vi "Image_Slider.vi"() -> ()   [LabVIEW 2016]
panel:
  out "2D Picture":picture
  in  "Folder of Images":path
  in  "Timeout":i32=100
  in  "Slide through your images":i32(slide) max=101 scale=0.0..100.0
  in  "OK":bool
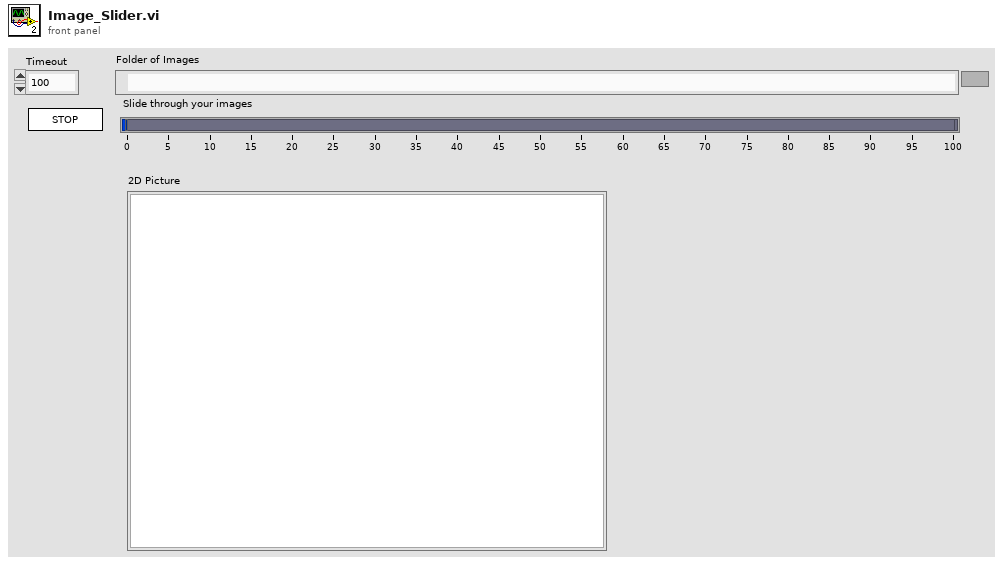
[diagram p1: front panel]
types:
  T1 = enum32{"invalid app kind", "Development System", "Run Time System", "Student Edition", "Embedded LabVIEW", "Evaluation", "Custom"}
  T2 = enum32{"Invalid", "Standard", "Closed", "Hidden", "Minimized", "Maximized"}
  T3 = cluster{"Core":cluster{"Current VI Reference":refnum<vi>, "Close Panel on Exit?":bool}, "Your Boolean data":bool, "Your string data":string, picture[], "individual picture":picture, "Folder of Images":path, i32, i32}
  T4 = cluster{"Current VI Reference":refnum<vi>, "Close Panel on Exit?":bool}
  T5 = typedef "imagedata.ctl" = cluster{"image type":i32, "image depth":i32, "image":u8[], "mask":u8[], "colors":u32[], "Rectangle":cluster{"left":i16, "top":i16, "right":i16, "bottom":i16}}
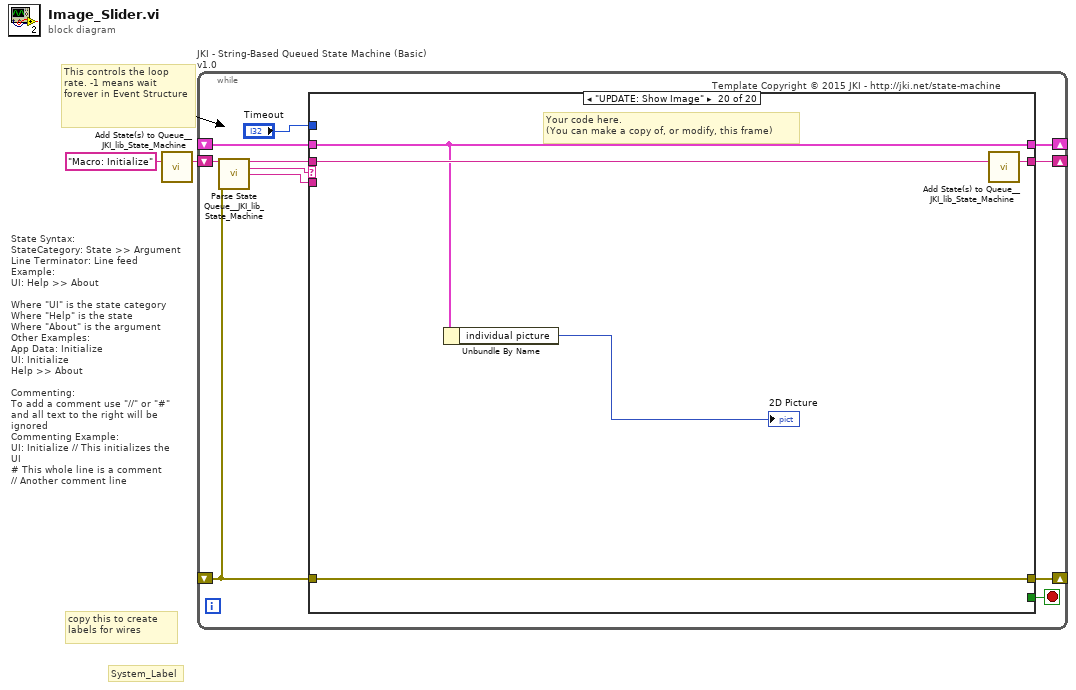
[diagram p0: block diagram]
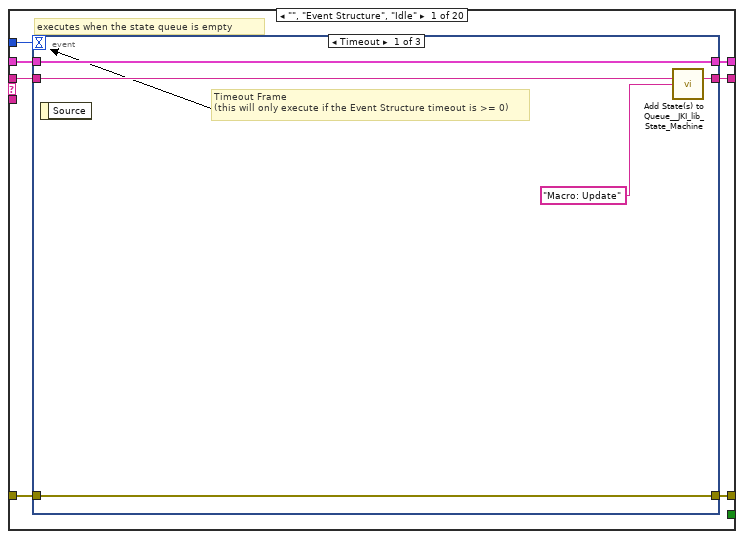
[diagram p2: hidden frame]
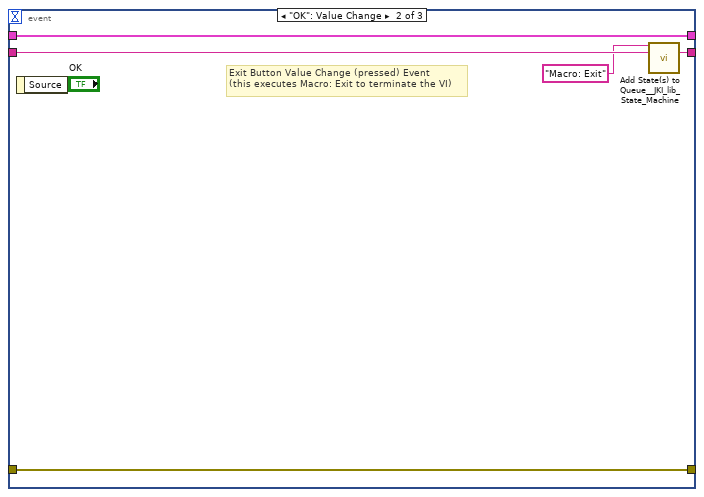
[diagram p3: hidden frame]
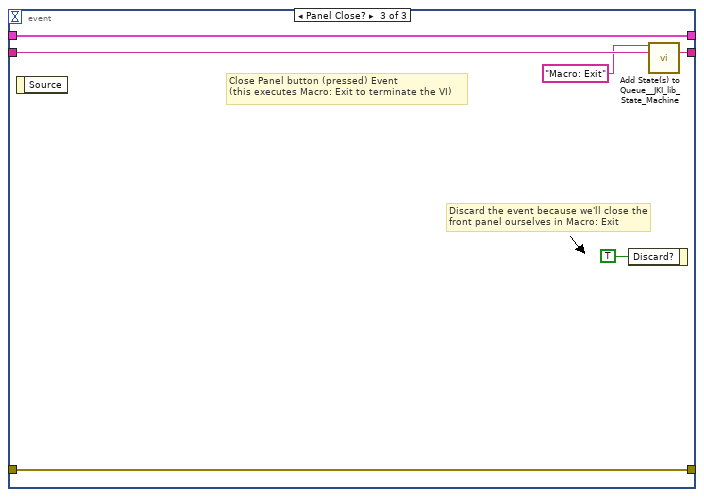
[diagram p4: hidden frame]
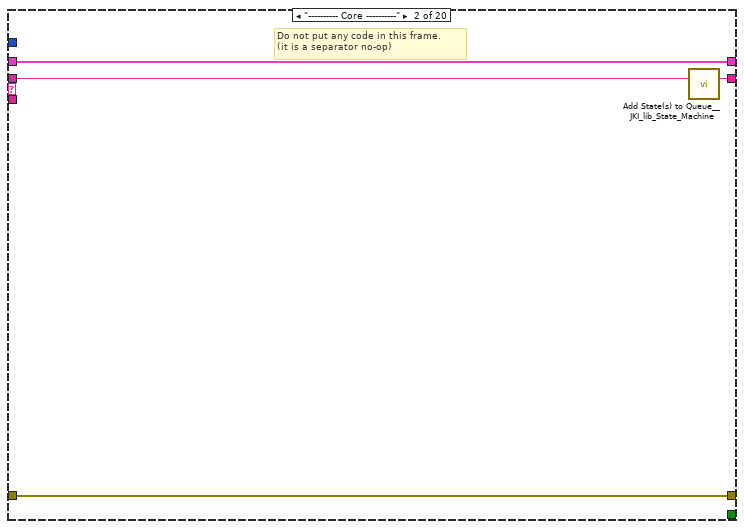
[diagram p5: hidden frame]
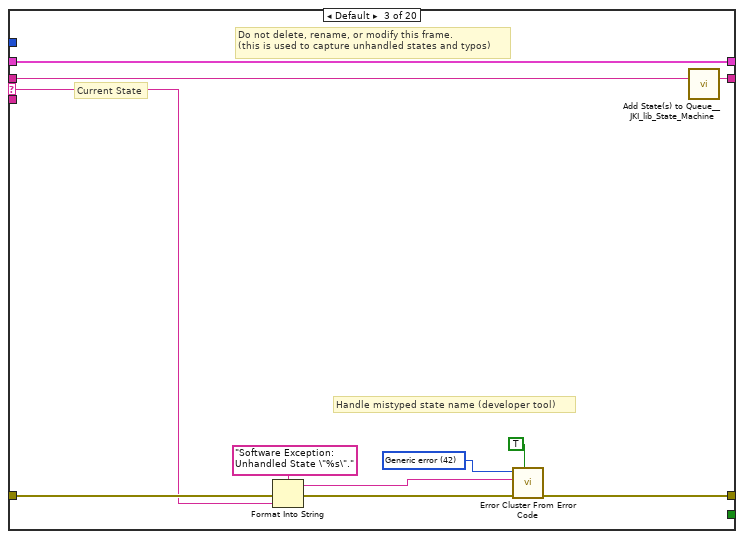
[diagram p6: hidden frame]
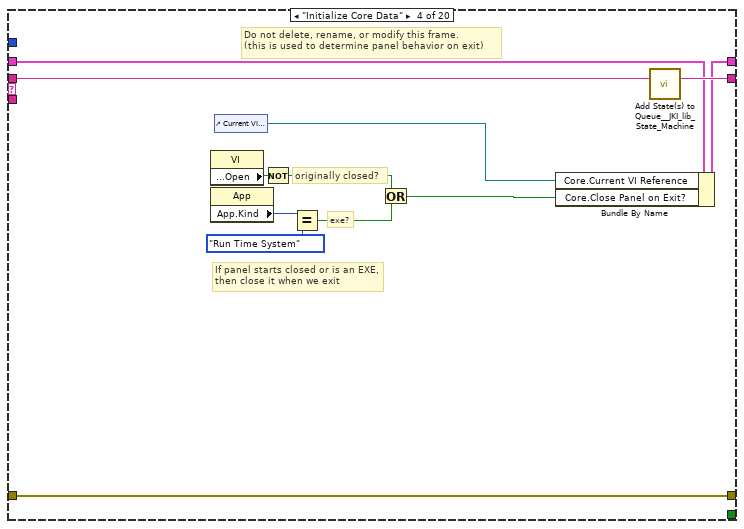
[diagram p7: hidden frame]
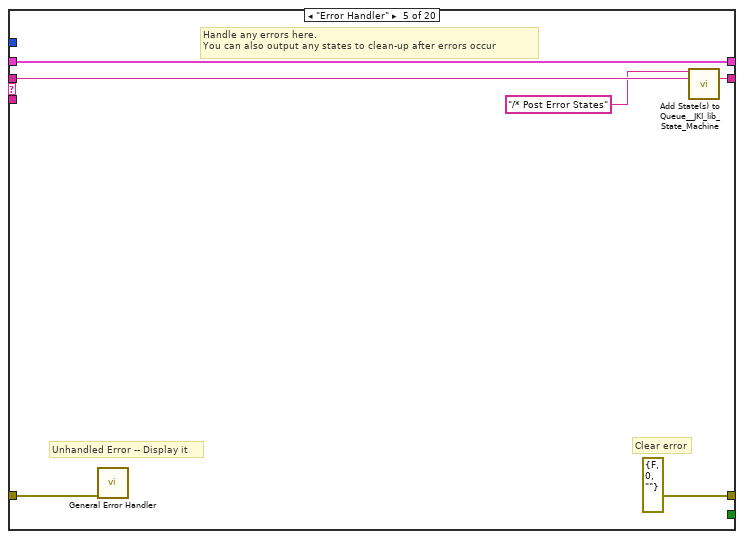
[diagram p8: hidden frame]
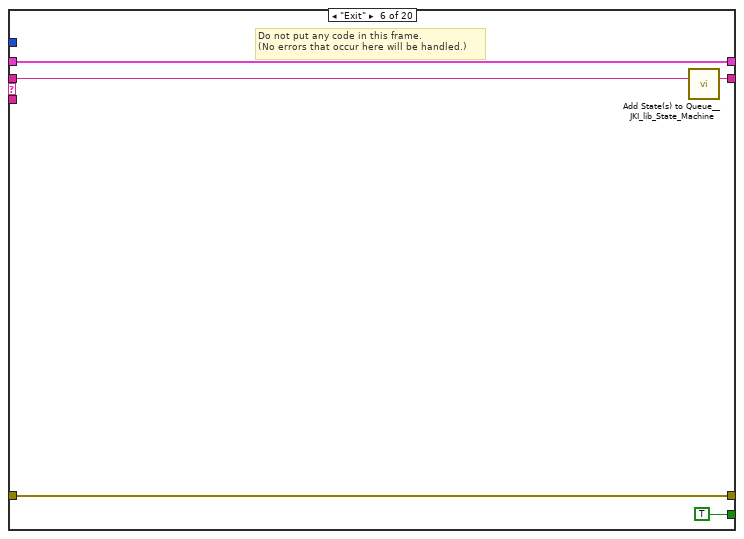
[diagram p9: hidden frame]
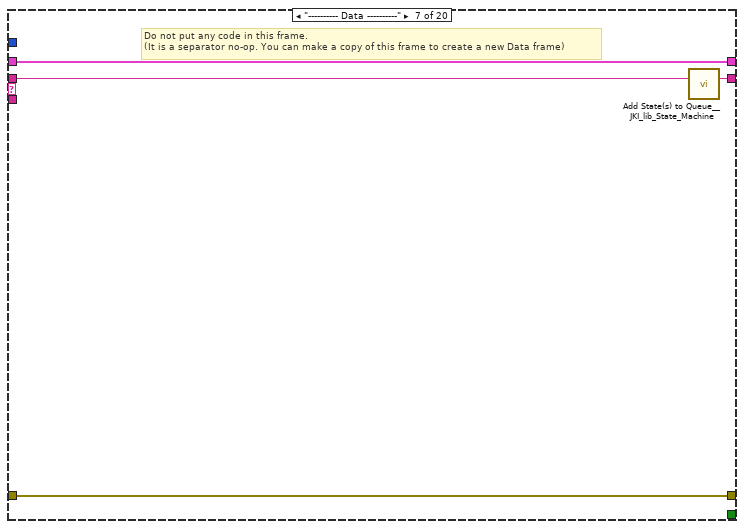
[diagram p10: hidden frame]
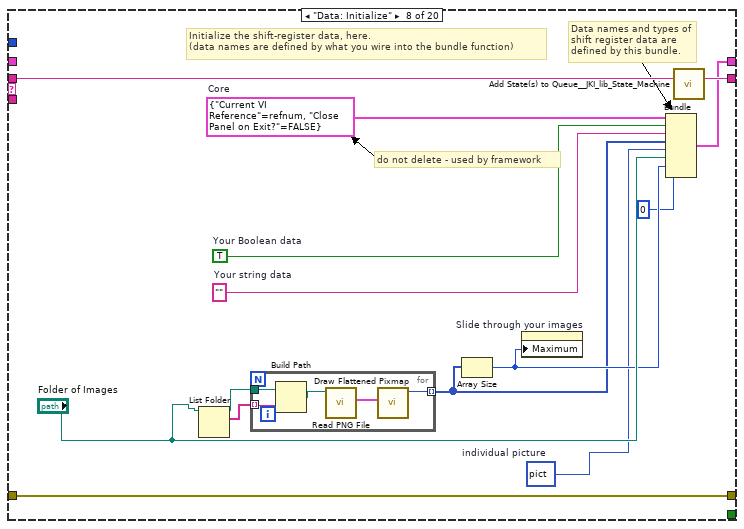
[diagram p11: hidden frame]
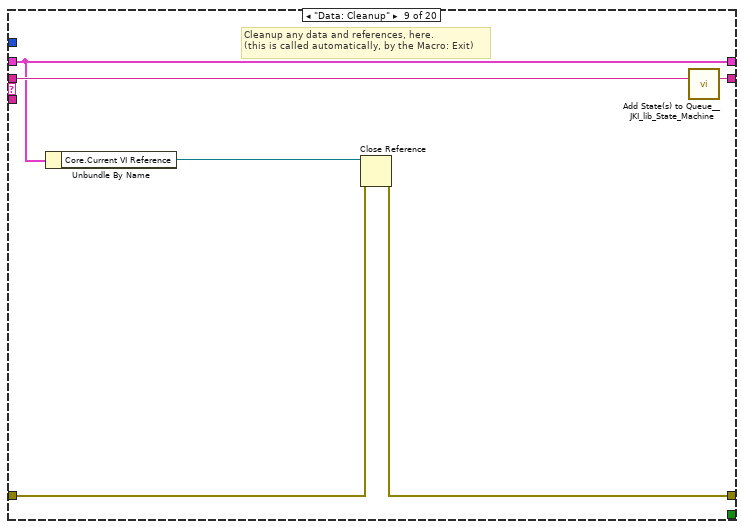
[diagram p12: hidden frame]
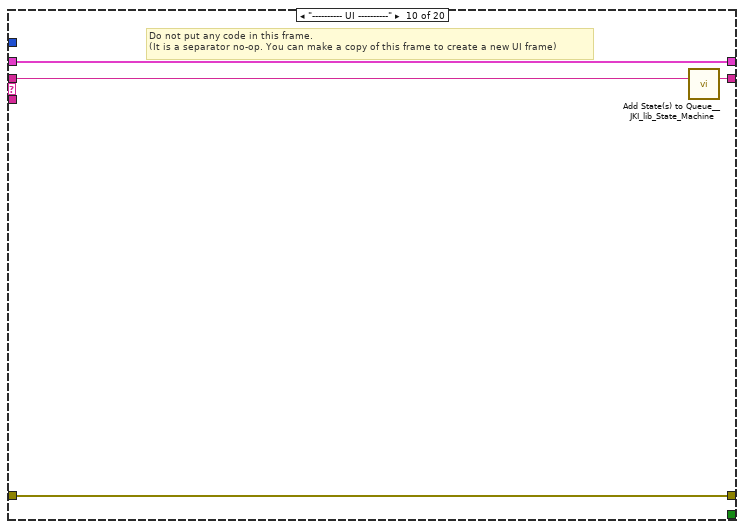
[diagram p13: hidden frame]
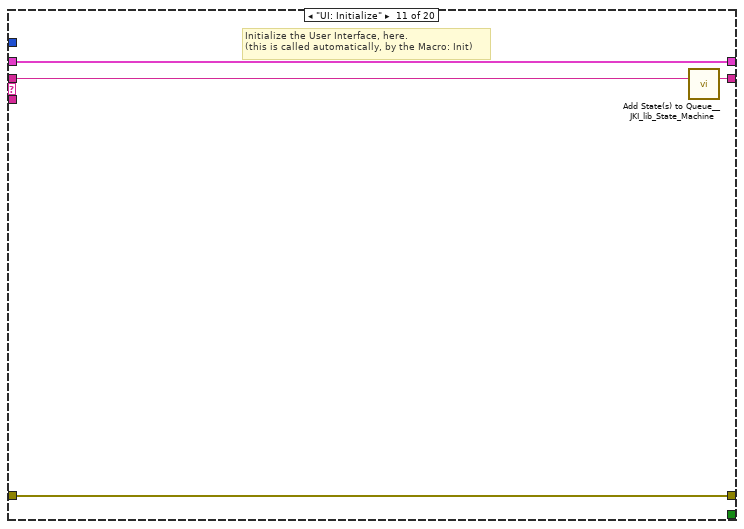
[diagram p14: hidden frame]
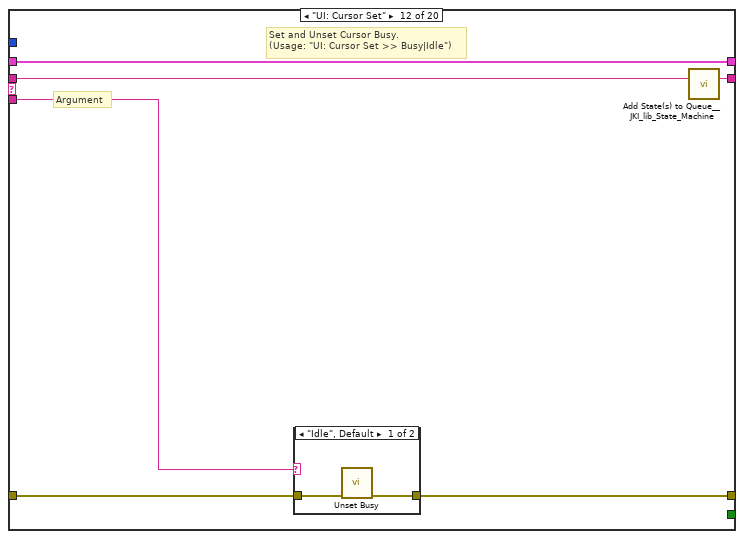
[diagram p15: hidden frame]
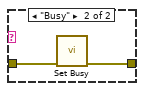
[diagram p16: hidden frame]
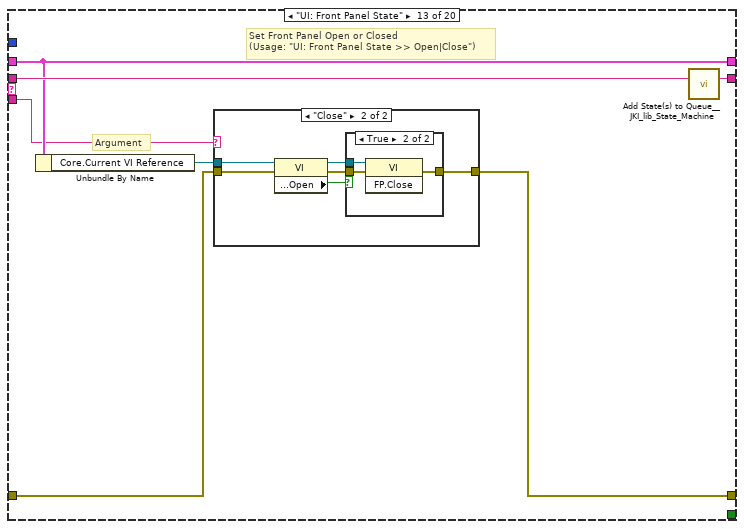
[diagram p17: hidden frame]
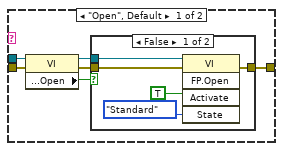
[diagram p18: hidden frame]
diagram:
  # "State Syntax:\nStateCategory: State >> Argument\nLine Terminator: Line feed\nExample:\nUI: Help >> About\n\nWhere \"UI\" is the state category\nWhere \"Help\" is the state\nWhere \"About\" is the argument\nOther Examples:\nApp Data: Initialize\nUI: Initialize\nHelp >> About\n\nCommenting:\nTo add a comment use \"//\" or \"#\" and all text to the right will be ignored\nCommenting Example:\nUI: Initialize // This initializes the UI\n# This whole line is a comment\n// Another comment line"
  # "copy this to create labels for wires"
  # "This controls the loop rate. -1 means wait forever in Event Structure"
  # "System_Label"
  n1 = call <vilib>:"Add State(s) to Queue__JKI_lib_State_Machine.vi"("State(s) in (\"\")"="Macro: Initialize") -> ("States Out"=w2:string)  [unwired: 14 in]
  n2 = while "JKI - String-Based Queued State Machine (Basic) v1.0" {
    shift-right: [w6] -> _
    shift-left: _ -> [w5]
    shift-right: [w9] -> _
    shift-left: _ -> [w3]
    shift-right: [w8] -> _
    shift-left: w2 -> [w10]
    stop <- w7 stop-if-true
    # "Template Copyright © 2015 JKI - http://jki.net/state-machine"
    n3 = call <vilib>:"Parse State Queue__JKI_lib_State_Machine.vi"("State Queue"=w10, "Error In (no error)"=w3) -> ("Remaining States"=w12:string, "Current State"=w13:string, "Arguments"=w11:string)  [unwired: 11 in]
    n4 = case shown="\"UPDATE: Show Image\"" w13 {
      selector: w13 -> [_ _ w41 _ _ _ _ _ _ _ _ _ _ _ _ _ _ _ _ _]
      tunnel: w12 -> [w20 w40 w45 w63 w69 w74 w78 w92 w103 w107 w111 w117 w128 w154 w159 w169 w174 w178 w186 w191]
      tunnel: w11 -> [_ _ _ _ _ _ _ _ _ _ _ w112 w122 _ _ _ _ _ _ _]
      tunnel: w5 -> [w18 w37 w43 w54 w66 w72 w75 _ w98 w104 w109 w115 w124 w151 w156 w166 w171 w175 w181 w188]
      tunnel: [w17 w38 w47 w60 errorcluster {"status"=FALSE, "code"=0, "source"=""} ("error out") w71 w76 w89 w99 w105 w108 w113 w125 w152 w157 w167 w172 w176 w184 w189] -> w9
      tunnel: w3 -> [w16 w38 w46 w60 w65 w71 w76 w89 w100 w105 w108 w114 w126 w152 w157 w167 w172 w176 w184 w189]
      tunnel: [w19 w39 w44 w62 w68 w73 w77 w91 w102 w106 w110 w116 w127 w153 w158 w168 w173 w177 w185 w190] -> w8
      tunnel: [_ _ _ _ _ TRUE _ _ _ _ _ _ _ _ _ _ _ _ _ _] -> w7
      tunnel: [w15 w37 w43 w61 w66 w72 w75 w90 w98 w104 w109 w115 w124 w151 w156 w166 w171 w175 w182 w188] -> w6
      tunnel: "Timeout" -> [w14 _ _ _ _ _ _ _ _ _ _ _ _ _ _ _ _ _ _ _]
      frame "", "Event Structure", "Idle" {
        # "executes when the state queue is empty"
        n5 = event shown="[0] Timeout" {
          selector: _ -> [_ _ _]
          dyn-events: _ -> [_ _ _]
          timeout: w14 -> [_ _ _]
          tunnel: w20 -> [w25 w30 w36]
          tunnel: [w24 w29 w35] -> w19
          tunnel: w18 -> [w22 w27 w33]
          tunnel: [w23 w28 w34] -> w17
          tunnel: w16 -> [w23 w28 w34]
          tunnel: [w22 w27 w33] -> w15
          event Timeout {
            # "Timeout Frame\n(this will only execute if the Event Structure timeout is >= 0)"
            n6 = event-data() -> ()  [unwired: 1 in, 1 out]
            n7 = call <vilib>:"Add State(s) to Queue__JKI_lib_State_Machine.vi"("State(s) in (\"\")"=w25, "State(s) at Back (\"\")"="Macro: Update" ("State(s) at Back (\"\")")) -> ("States Out"=w24:string)  [unwired: 13 in]
          }
          event "OK": Value Change {
            # "Exit Button Value Change (pressed) Event\n(this executes Macro: Exit to terminate the VI)"
            n8 = event-data() -> ()  [unwired: 1 in, 1 out]
            n9 = call <vilib>:"Add State(s) to Queue__JKI_lib_State_Machine.vi"("State(s) in Front (\"\")"="Macro: Exit", "State(s) in (\"\")"=w30) -> ("States Out"=w29:string)  [unwired: 13 in]
          }
          event Panel Close? {
            # "Discard the event because we'll close the front panel ourselves in Macro: Exit"
            # "Close Panel button (pressed) Event\n(this executes Macro: Exit to terminate the VI)"
            n10 = event-data() -> ()  [unwired: 1 in, 1 out]
            n11 = event-data("Discard?"=TRUE) -> ()  [unwired: 1 in, 1 out]
            n12 = call <vilib>:"Add State(s) to Queue__JKI_lib_State_Machine.vi"("State(s) in Front (\"\")"="Macro: Exit", "State(s) in (\"\")"=w36) -> ("States Out"=w35:string)  [unwired: 13 in]
          }
        }
      }
      frame "---------- Core ----------" {
        # "Do not put any code in this frame.\n(it is a separator no-op)"
        n13 = call <vilib>:"Add State(s) to Queue__JKI_lib_State_Machine.vi"("State(s) in (\"\")"=w40) -> ("States Out"=w39:string)  [unwired: 14 in]
      }
      frame Default {
        w50 = 42 items=["No error", "Argument error", "Memory is full", "Out of zone", "End of file", "File already open", "Generic file I/O error", "File not found", "File permission error", "Disk is full", "Duplicate path", "Too many files open", "System feature not enabled", "Resource file not found", "Cannot add resource", "Resource not found", "Image not found", "Image memory error", "Pen does not exist", "Config type invalid", "Config token not found", "Config parse error", "Config memory error", "Bad external code format", "Bad external code offset", "External code not present", "Null window", "Destroy window error", "Null menu", "Print aborted", "Bad print record", "Print driver error", "Windows error during printing", "Memory error during printing", "Print dialog error", "Generic print error", "Invalid device refnum", "Device not found", "Device parameter error", "Device unit error", "Cannot open device", "Device call aborted", "Generic error", "Cancelled by user", "Object ID too low", "Object ID too high", "Object not in heap", "Unknown heap", "Unknown object (invalid DefProc)", "Unknown object (DefProc not in table)", "Message out of range", "Invalid (null) method", "Unknown message", "Manager call not supported", "Bad address", "Network operation in progress", "Network operation timed out", "Connection is busy", "Network attribute not supported", "Network error", "Address in use", "System out of memory", "Connection aborted", "Connection refused", "Not connected", "Already connected", "Connection closed", "Initialization error (interapplication manager)", "Bad occurrence", "Wait on unbound occurrence handler", "Occurrence queue overflow", "Datalog type conflict", "Unused", "Unrecognized type (interapplication manager)", "Memory corrupt", "Failed to make temporary DLL", "Old CIN version", "Drag socket not found", "Failed to load drop-object", "Failed to register OLE object", "Failed to release OLE object", "Format specifier type mismatch", "Unknown format specifier", "Too few format specifiers", "Too many format specifiers", "Scan failed", "Newer CIN version", "Error converting to variant", "Runtime menu error", "Password tampered", "Variant attribute not found", "Incompatible variant data type", "Event data is not available", "Event Store is not present", "Occurrence is not found", "Event Queue is not created", "Event info is not available", "Refnum passed is NULL", "Error retrieving Class GUID", "Error retrieving CoClass GUID", "Error retrieving TypeLib GUID.", "Bad built application magic bytes.", "Specific driver is different from the specific driver associated with the Logical Name.", "There is no session opened to the class driver.", "Max Error", "MAX - Error with config objects", "MAX - Error loading configuration", "MAX - Group not supported"]
        # "Current State"
        # "Do not delete, rename, or modify this frame.\n(this is used to capture unhandled states and typos)"
        # "Handle mistyped state name (developer tool)"
        n14 = Format Into String(format string="Software Exception: Unhandled State \"%s\"." ("message"), error in=w46, w41) -> (resulting string=w49:string, error out=w48:errorcluster)  [unwired: 1 in]
        n15 = call <vilib>:"Error Cluster From Error Code.vi"("show call chain? (False)"=TRUE, "error in (no error)"=w48, "error message (\"\")"=w49, "error code (0)"=w50) -> ("error out"=w47:errorcluster)  [unwired: 5 in]
        n16 = call <vilib>:"Add State(s) to Queue__JKI_lib_State_Machine.vi"("State(s) in (\"\")"=w45) -> ("States Out"=w44:string)  [unwired: 14 in]
      }
      frame "Initialize Core Data" {
        # "Do not delete, rename, or modify this frame.\n(this is used to determine panel behavior on exit)"
        # "originally closed?"
        # "exe?"
        # "If panel starts closed or is an EXE, then close it when we exit"
        n17 = property class="VI"() -> ("Front Panel.Open"=w59:bool)  [unwired: 2 in, 2 out]
        n18 = property class="App"() -> ("App.Kind"=w58:T1)  [unwired: 2 in, 2 out]
        n19 = control-ref of="Current VI Reference"() -> (w52:refnum<vi>)
        n20 = Not(x=w59) -> (.not. x?=w56:bool)
        n21 = Equal?(x=w58, y=T1."Run Time System" ("Application:Kind")) -> (x = y?=w55:bool)
        n22 = Or(x=w56, y=w55) -> (x .or. y?=w53:bool)
        n23 = Bundle By Name(cluster=w54, "Core.Current VI Reference"=w52, "Core.Close Panel on Exit?"=w53) -> (w61:T3)
        n24 = call <vilib>:"Add State(s) to Queue__JKI_lib_State_Machine.vi"("State(s) in (\"\")"=w63) -> ("States Out"=w62:string)  [unwired: 14 in]
      }
      frame "Error Handler" {
        # "Unhandled Error -- Display it"
        # "Handle any errors here.\nYou can also output any states to clean-up after errors occur"
        # "Clear error"
        n25 = call <vilib>:"General Error Handler.vi"("error in (no error)"=w65) -> ()  [unwired: 10 in, 5 out]
        n26 = call <vilib>:"Add State(s) to Queue__JKI_lib_State_Machine.vi"("State(s) in Front (\"\")"="/* Post Error States", "State(s) in (\"\")"=w69) -> ("States Out"=w68:string)  [unwired: 13 in]
      }
      frame "Exit" {
        # "Do not put any code in this frame.\n(No errors that occur here will be handled.)"
        n27 = call <vilib>:"Add State(s) to Queue__JKI_lib_State_Machine.vi"("State(s) in (\"\")"=w74) -> ("States Out"=w73:string)  [unwired: 14 in]
      }
      frame "---------- Data ----------" {
        # "Do not put any code in this frame.\n(It is a separator no-op. You can make a copy of this frame to create a new Data frame)"
        n28 = call <vilib>:"Add State(s) to Queue__JKI_lib_State_Machine.vi"("State(s) in (\"\")"=w78) -> ("States Out"=w77:string)  [unwired: 14 in]
      }
      frame "Data: Initialize" {
        w81 = picture data[5B]  # individual picture
        w86 = T4 {"Current VI Reference"=refnum, "Close Panel on Exit?"=FALSE}  # Core
        w88 = TRUE  # Your Boolean data
        w87 = ""  # Your string data
        # "do not delete - used by framework"
        # "Data names and types of shift register data are defined by this bundle."
        # "Initialize the shift-register data, here.\n(data names are defined by what you wire into the bundle function)"
        n29 = List Folder(path="Folder of Images") -> (path out=w82:path, filenames=w83:string[])  [unwired: 3 in, 2 out]
        n30 = for {
          tunnel: w83 -> [w95] mode=indexing
          tunnel: w82 -> [w94]
          tunnel: [w93] -> w79 mode=indexing
          n31 = Build Path(base path=w94, name or relative path=w95) -> (appended path=w97:path)
          n32 = call <vilib>:"Read PNG File.vi"("path to PNG file"=w97) -> ("image data"=w96:T5)  [unwired: 8 in, 2 out]
          n33 = call <vilib>:"Draw Flattened Pixmap.vi"("image data"=w96) -> ("new picture"=w93:picture)  [unwired: 8 in]
        }
        n34 = Array Size(array=w79) -> (size(s)=w84:i32)
        n35 = property on="Slide through your images" class="Slide (strict)"("Maximum"=w84) -> ()  [unwired: 2 in, 2 out]
        n36 = Bundle("Core"=w86, "Your Boolean data"=w88, "Your string data"=w87, w79, "individual picture"=w81, "Folder of Images"="Folder of Images", w84, 0) -> (w90:T3)  [unwired: 1 in]
        n37 = call <vilib>:"Add State(s) to Queue__JKI_lib_State_Machine.vi"("State(s) in (\"\")"=w92) -> ("States Out"=w91:string)  [unwired: 14 in]
      }
      frame "Data: Cleanup" {
        # "Cleanup any data and references, here.\n(this is called automatically, by the Macro: Exit)"
        n38 = Unbundle By Name(w98) -> ("Core.Current VI Reference"=w101:refnum<vi>)
        n39 = Close Reference(reference=w101, error in (no error)=w100) -> (error out=w99:errorcluster)
        n40 = call <vilib>:"Add State(s) to Queue__JKI_lib_State_Machine.vi"("State(s) in (\"\")"=w103) -> ("States Out"=w102:string)  [unwired: 14 in]
      }
      frame "---------- UI ----------" {
        # "Do not put any code in this frame.\n(It is a separator no-op. You can make a copy of this frame to create a new UI frame)"
        n41 = call <vilib>:"Add State(s) to Queue__JKI_lib_State_Machine.vi"("State(s) in (\"\")"=w107) -> ("States Out"=w106:string)  [unwired: 14 in]
      }
      frame "UI: Initialize" {
        # "Initialize the User Interface, here.\n(this is called automatically, by the Macro: Init)"
        n42 = call <vilib>:"Add State(s) to Queue__JKI_lib_State_Machine.vi"("State(s) in (\"\")"=w111) -> ("States Out"=w110:string)  [unwired: 14 in]
      }
      frame "UI: Cursor Set" {
        # "Argument"
        # "Set and Unset Cursor Busy.\n(Usage: \"UI: Cursor Set >> Busy|Idle\")"
        n43 = case shown="\"Idle\", Default" w112 {
          tunnel: w114 -> [w119 w121]
          tunnel: [w118 w120] -> w113
          frame "Idle", Default {
            n44 = call <vilib>:"Unset Busy.vi"("error in (no error)"=w119) -> ("error out"=w118:errorcluster)  [unwired: 10 in]
          }
          frame "Busy" {
            n45 = call <vilib>:"Set Busy.vi"("error in (no error)"=w121) -> ("error out"=w120:errorcluster)  [unwired: 9 in, 1 out]
          }
        }
        n46 = call <vilib>:"Add State(s) to Queue__JKI_lib_State_Machine.vi"("State(s) in (\"\")"=w117) -> ("States Out"=w116:string)  [unwired: 14 in]
      }
      frame "UI: Front Panel State" {
        # "Argument"
        # "Set Front Panel Open or Closed\n(Usage: \"UI: Front Panel State >> Open|Close\")"
        n47 = Unbundle By Name(w124) -> ("Core.Current VI Reference"=w123:refnum<vi>)
        n48 = case shown="\"Close\"" w122 {
          tunnel: w126 -> [w132 w145]
          tunnel: [w134 w146] -> w125
          tunnel: w123 -> [w133 w143]
          frame "Open", Default {
            n49 = property class="VI"(reference=w133, error in=w132) -> (reference out=w130:refnum<vi>, error out=w131:errorcluster, "Front Panel.Open"=w129:bool)
            n50 = case shown="False" w129 {
              tunnel: [w137 w140] -> w134
              tunnel: w131 -> [w136 w140]
              tunnel: w130 -> [w135 _]
              frame False {
                n51 = invoke class="VI" method="FP.Open"(reference=w135, error in=w136, "Activate"=TRUE, "State"=T2."Standard") -> (error out=w137:errorcluster)  [unwired: 1 in, 4 out]
              }
              frame True {
              }
            }
          }
          frame "Close" {
            n52 = property class="VI"(reference=w143, error in=w145) -> (reference out=w142:refnum<vi>, error out=w144:errorcluster, "Front Panel.Open"=w141:bool)
            n53 = case shown="True" w141 {
              tunnel: [w147 w150] -> w146
              tunnel: w144 -> [w147 w149]
              tunnel: w142 -> [_ w148]
              frame False {
              }
              frame True {
                n54 = invoke class="VI" method="FP.Close"(reference=w148, error in=w149) -> (error out=w150:errorcluster)  [unwired: 1 in, 2 out]
              }
            }
          }
        }
        n55 = call <vilib>:"Add State(s) to Queue__JKI_lib_State_Machine.vi"("State(s) in (\"\")"=w128) -> ("States Out"=w127:string)  [unwired: 14 in]
      }
      frame "---------- Macro ----------" {
        # "Do not put any code in this frame.\n(It is a separator no-op. You can make a copy of this frame to create a new Macro frame)"
        n56 = call <vilib>:"Add State(s) to Queue__JKI_lib_State_Machine.vi"("State(s) in (\"\")"=w154) -> ("States Out"=w153:string)  [unwired: 14 in]
      }
      frame "Macro: Initialize" {
        w155 = "Data: Initialize\nInitialize Core Data\nUI: Initialize\nUI: Front Panel State >> Open"  # Data: Initialize Initialize Core Data UI: Initialize UI: Front Panel State >> Open
        # "Initialization Macro\n(This is called once, when the VI starts)"
        n57 = call <vilib>:"Add State(s) to Queue__JKI_lib_State_Machine.vi"("State(s) in Front (\"\")"=w155, "State(s) in (\"\")"=w159) -> ("States Out"=w158:string)  [unwired: 13 in]
      }
      frame "Macro: Exit" {
        # "Exit Macro\n(This is called once, when the VI exits)"
        n58 = Unbundle By Name(w166) -> ("Core.Close Panel on Exit?"=w165:bool)
        n59 = Select(t="UI: Front Panel State >> Close", s=w165, f="") -> (s? t:f=w162:string)
        n60 = call <vilib>:"Add State(s) to Queue__JKI_lib_State_Machine.vi"("State(s) in (\"\")"=w162, "State(s) at Back (\"\")"="Data: Cleanup\nExit") -> ("States Out"=w160:string)  [unwired: 13 in]
        n61 = call <vilib>:"Add State(s) to Queue__JKI_lib_State_Machine.vi"("State(s) in Front (\"\")"=w160, "State(s) in (\"\")"=w169) -> ("States Out"=w168:string)  [unwired: 13 in]
      }
      frame "Macro: Update" {
        # "Exit Macro\n(This is called once, when the VI exits)"
        n62 = call <vilib>:"Add State(s) to Queue__JKI_lib_State_Machine.vi"("State(s) in Front (\"\")"="UPDATE: Select Image\nUPDATE: Show Image", "State(s) in (\"\")"=w174) -> ("States Out"=w173:string)  [unwired: 13 in]
      }
      frame "---------- UPDATE ----------" {
        # "Template Separator\n(You can make a copy of, or modify, this frame)"
        n63 = call <vilib>:"Add State(s) to Queue__JKI_lib_State_Machine.vi"("State(s) in (\"\")"=w178) -> ("States Out"=w177:string)  [unwired: 14 in]
      }
      frame "UPDATE: Select Image" {
        n64 = Unbundle(w181) -> (w180:picture[])  [unwired: 7 out]
        n65 = Index Array(array=w180, index="Slide through your images") -> (element=w179:picture)
        n66 = Bundle By Name(cluster=w181, "individual picture"=w179) -> (w182:T3)
        n67 = call <vilib>:"Add State(s) to Queue__JKI_lib_State_Machine.vi"("State(s) in (\"\")"=w186) -> ("States Out"=w185:string)  [unwired: 14 in]
      }
      frame "UPDATE: Show Image" {
        # "Your code here.\n(You can make a copy of, or modify, this frame)"
        n68 = Unbundle By Name(w188) -> ("individual picture"=→"2D Picture":picture)
        n69 = call <vilib>:"Add State(s) to Queue__JKI_lib_State_Machine.vi"("State(s) in (\"\")"=w191) -> ("States Out"=w190:string)  [unwired: 14 in]
      }
    }
  }
